vi "Modify name 03-ddT.vi"(0 "path":path=path "F:/fh/传输D/2015谷粒实验/提取数据/后期处理数据/3-总反射率 二阶") -> ()   [LabVIEW 2015]
uses:
  <vilib>/Utility/file.llb/Read Delimited Spreadsheet (string).vi
  <vilib>/Utility/file.llb/Write Delimited Spreadsheet (string).vi
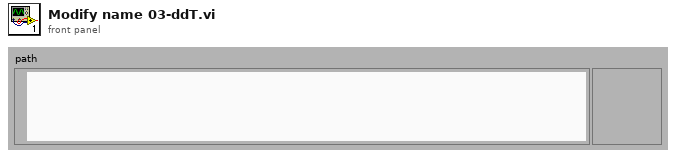
[diagram p1: front panel]
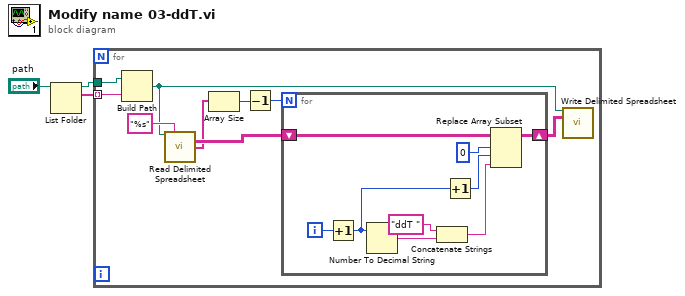
[diagram p0: block diagram]
diagram:
  n1 = List Folder(path="path") -> (path out=w1:path, filenames=w2:string[])  [unwired: 1 in, 4 out]
  n2 = for {
    tunnel: w2 -> [w11] mode=indexing
    tunnel: w1 -> [w12]
    n3 = Build Path(base path=w12, name or relative path=w11) -> (appended path=w6:path)
    n4 = call-poly <vilib>:"Read Delimited Spreadsheet.vi"("file path (dialog if empty)"=w6, "format (%s)"="%s") -> ("all rows"=w7:string[][], "first row"=w5:string[])  [unwired: 8 in, 4 out]
    n5 = Array Size(array=w5) -> (size(s)=w9:i32)
    n6 = Decrement(x=w9) -> (x-1=w8:i32)
    n7 = for {
      N: w8 -> [_]
      shift-right: [w15] -> w4
      shift-left: w7 -> [w21]
      i -> [w19]
      n8 = Increment(x=w19) -> (x+1=w14:i32)
      n9 = Number To Decimal String(number=w14) -> (decimal integer string=w18:string)  [unwired: 1 out]
      n10 = Concatenate Strings("ddT " ("string"), w18) -> (w16:string)
      n11 = Increment(x=w14) -> (x+1=w13:i32)
      n12 = Replace Array Subset(array=w21, new element=w16, index (row)=0, index (col)=w13) -> (w15:string[][])
    }
    n13 = call-poly <vilib>:"Write Delimited Spreadsheet.vi"("file path (dialog if empty)"=w6, "2D data"=w4) -> ()  [unwired: 12 in, 2 out]
  }
